vi "Load actor by relative path.vi"(8 "error in (no error)":errorcluster, 11 "Path":string) -> (0 "error out":errorcluster, 3 "Actor":refnum<class "Actor.lvclass">)   [LabVIEW 2014]
uses:
  <vilib>/ActorFramework/Actor/Actor.lvclass
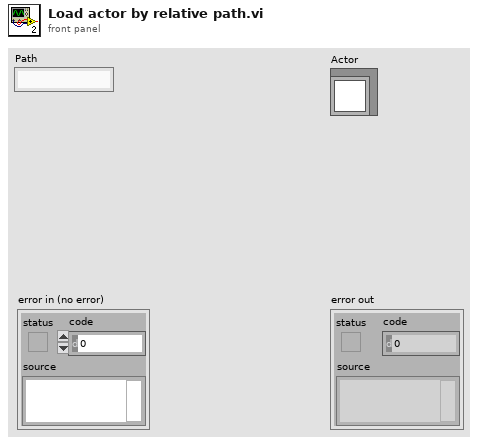
[diagram p1: front panel]
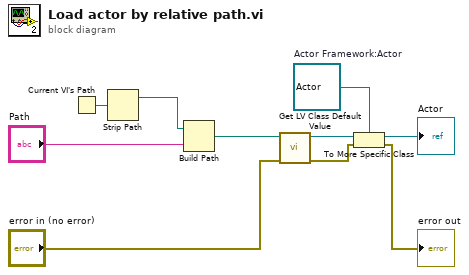
[diagram p0: block diagram]
diagram:
  w4 = refnum<class "Actor.lvclass"> refnum  # Actor Framework:Actor
  n1 = Current VI's Path() -> (path=w10:path)
  n2 = Strip Path(path=w10) -> (stripped path=w9:path)  [unwired: 1 out]
  n3 = Build Path(base path=w9, name or relative path="Path") -> (appended path=w7:path)
  n4 = call <vilib>:"Get LV Class Default Value.vi"("error in (no error)"="error in (no error)", "class path"=w7) -> ("error out"=w5:errorcluster, "object"=w6:refnum<class>)  [unwired: 8 in]
  n5 = To More Specific Class(target class=w4, reference=w6, error in=w5) -> (specific class reference=→"Actor":refnum<class "Actor.lvclass">, error out=→"error out":errorcluster)
